vi "getLocalRepoVersions.vi"(8 "error in (no error)":errorcluster, 11 "repoHandlers in":refnum<class "repoHandler.lvclass">[](array[class])) -> (0 "error out":errorcluster, 3 "repoHandlers":refnum<class "repoHandler.lvclass">[](array[class]))   [LabVIEW 2013]
uses:
  repoHandler/repoHandler.lvclass
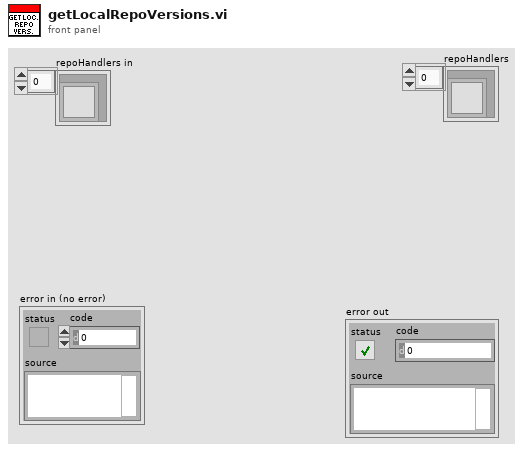
[diagram p1: front panel]
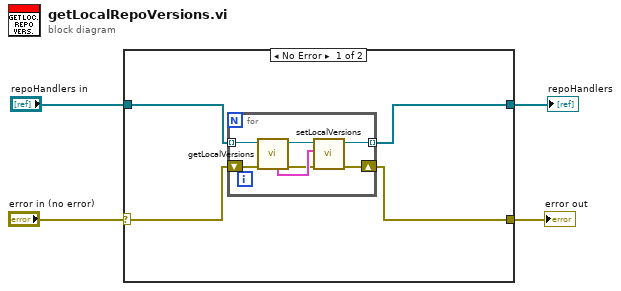
[diagram p0: block diagram]
diagram:
  n1 = case shown="No Error" "error in (no error)" {
    selector: "error in (no error)" -> [w6 w16]
    tunnel: [w5 w16] -> w3
    tunnel: "repoHandlers in" -> [w8 w17]
    tunnel: [w7 w17] -> w1
    frame No Error {
      n2 = for {
        tunnel: w8 -> [w15] mode=indexing
        tunnel: [w13] -> w7 mode=indexing
        shift-right: [w9] -> w5
        shift-left: w6 -> [w10]
        n3 = call-dynamic "getLocalVersions.vi"("error in (no error)"=w10, "repoHandler in"=w15) -> ("error out"=w11:errorcluster, "repoHandler out"=w14:refnum<class "repoHandler.lvclass">, "Local Versions"=w12:cluster{"version":string, "longHash":string}[])  [unwired: 7 in]
        n4 = call-dynamic "setLocalVersions.vi"("error in (no error)"=w11, "Local Versions"=w12, "repoHandler in"=w14) -> ("error out"=w9:errorcluster, "repoHandler out"=w13:refnum<class "repoHandler.lvclass">)  [unwired: 7 in]
      }
    }
    frame Error {
    }
  }
  "error out" <- w3
  "repoHandlers" <- w1
